vi "Right-Click - Template.vi"() -> ()   [LabVIEW 2011]
doc: "This display template will allow a user to add any numeric or boolean control or indicator to the front panel, and be able to configure it in VeriStand.\n\nSteps:\n1. Add Control / Indicator to the front panel\n2. Right-Click control / indicator and show the Caption (Visible Items >> Caption)\n**Note: No changes on the block diagram are required, however it is advised to put the new controls / indicators in the initialization portion of the code for continuity.\n3. Edit the VI front panel so it only shows the controls and thier captions.\n4. Change the VI window size (File >> VI Properties >> Window Size >> Set to Current)\n5. Save the VI, and Re-build the source distribution\n6. Place new source distribution files here: < Shared Documents >\\ National Instruments\\VeriStand\\Display Templates"
uses:
  <vilib>/NI Veristand/Display Template Support/Display Template Support.llb/cluster_Screen Item Settings.ctl
  <vilib>/NI Veristand/Display Template Support/Display Template Support.llb/cluster_Graph Scale Settings.ctl
  <vilib>/NI Veristand/Display Template Support/Display Template Support.llb/cluster_Graph Plot Settings.ctl
  NationalInstruments.VeriStand.SystemStorage
  <vilib>/NI Veristand/Display Template Support/Display Template Support.llb/enum_Display Template Handler Minimal To Widget Msg.ctl
  <vilib>/NI Veristand/Display Template Support/Display Template Support.llb/enum_Display Template Handler Minimal To Workspace.ctl
  Sub VIs/Custom Data Cluster Control.ctl
  <vilib>/NI Veristand/Display Template Support/Display Template Support.llb/sub_Display Template Handler Custom.vi
  <vilib>/NI Veristand/Execution/Workspace/NI VeriStand - Get Multiple Channel Values.vi
  <vilib>/NI Veristand/Execution/Workspace/NI VeriStand - Set Single Channel Value.vi
  <vilib>/NI Veristand/Execution/Workspace/NI_VS Workspace ExecutionAPI.lvlib
panel:
  in  "NIVS.System Definition Root":refnum<k24>
  in  "NIVS.Gateway IP Address":string
  in  "Ring":u16(ring) items=["Option 1", "Option 2", "Option 3"]
  in  "Boolean":bool
  out "error out":errorcluster
  out "Indicator 2":dbl caption="Numeric"
  out "Indicator 1":dbl caption="Numeric"
  in  "Control 2":dbl caption="Numeric"
  in  "Control 1":dbl caption="Numeric"
  in  "Item.Data":T1
  # "Right-Click a Control or Indicator to configure."
  # "This is needed for the channel selection dialog, do not modify"
  # "This is needed for multi host support, do not modify"
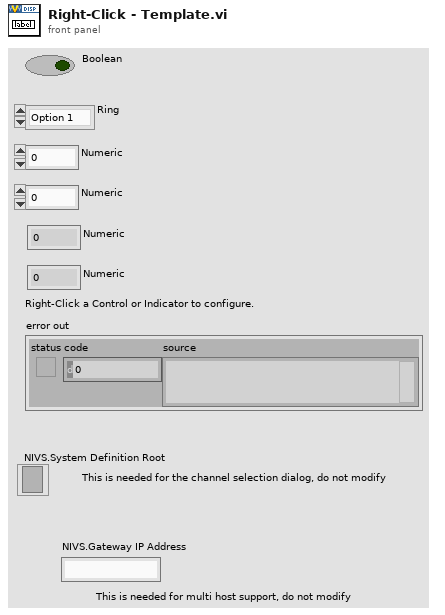
[diagram p1: front panel]
types:
  T1 = typedef "cluster_Screen Item Settings.ctl" = cluster{"Template VI":string, "Position X":i32, "Position Y":i32, "Custom":string, "Show Title Bar":bool, "ID":i32, "Always On Top":bool, "Allow Resize":bool, "Allow Minimize":bool, "Allow Close":bool, "Size to Screen":bool, "Screen.ID":i32, "State":enum16{"Normal", "New"}, "Title":string, "Window Bounds":cluster{"[0]":i16, "[1]":i16, "[2]":i16, "[3]":i16}, "Channel Ref":u64, "Unit":string, "Default Units?":bool, "Flash Limit?":bool, "Color 1":u32, "Color 2":u32, "Color 3":u32, "Color 4":u32, "Bck Color":u32, "Fore Color":u32, "Limit 1":dbl, "Limit 2":dbl, "Limit 3":dbl, "Limit 4":dbl, "Limit Mode 1":i32, "Limit Mode 2":i32, "Limit Mode 3":i32, "Limit Mode 4":i32, "Scale Precision":i32, "Scale Min":dbl, "Scale Max":dbl, "Format":i32, "Precision":i32, "Background Type":i32, "IDs":i32[], "Units":string[], "Labels":string[], "Scale Factor":dbl, "Scale Offset":dbl, "YScale Index":u32[], "XScale":T2, "YScales":T2[], "Plots":T3[], "Update Period":dbl, "History Length":dbl, "My.Ref":refnum<vi>, "Is Control?":bool, "Channel Paths":string[], "Custom Data":variant}
  T2 = typedef "cluster_Graph Scale Settings.ctl" = cluster{"Format":u8, "Precision":u8, "Fit":u8, "Label":string, "Use Default Label":bool, "Label Visible":bool, "Min":dbl, "Max":dbl}
  T3 = typedef "cluster_Graph Plot Settings.ctl" = cluster{"Bar Style":u8, "Fill To":i16, "Fill/PtColor":u32, "Line Style":u8, "Line Width":u8, "Color":u32, "Interp":u8, "Point Style":u8}
  T4 = typedef "enum_Display Template Handler Minimal To Workspace.ctl" = cluster{"Operation":enum16{"SetCustomData", "DeleteItem"}, "Data":variant}
  T5 = typedef "enum_Display Template Handler Minimal To Widget Msg.ctl" = enum16{"Stop", "LaunchConfigDialog"}
  T6 = typedef "Custom Data Cluster Control.ctl" = cluster{"All Refs":refnum<vi>[], "Paths":string[], "Indices":u32[], "NodePathArrays":string[][]}
  T7 = typedef "NI_VS Workspace ExecutionAPI.lvlib/WorkspaceAPI.ctl" = refnum<k24>
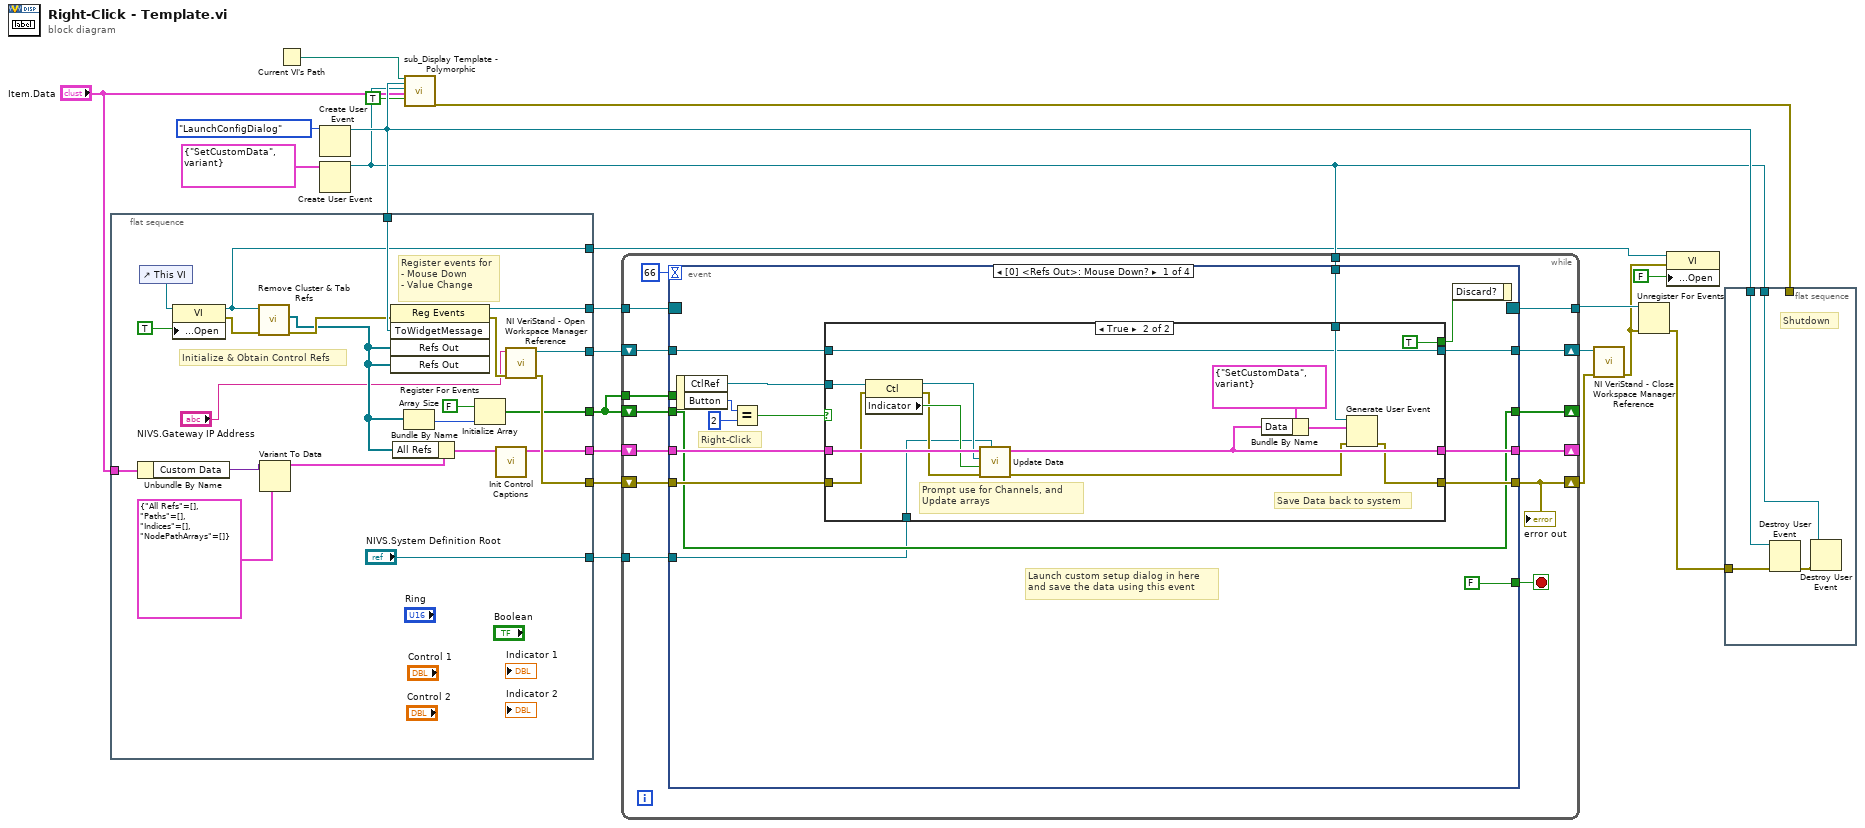
[diagram p0: block diagram]
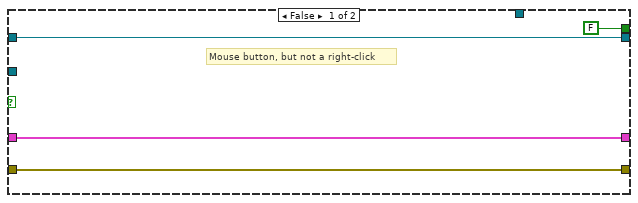
[diagram p2: hidden frame]
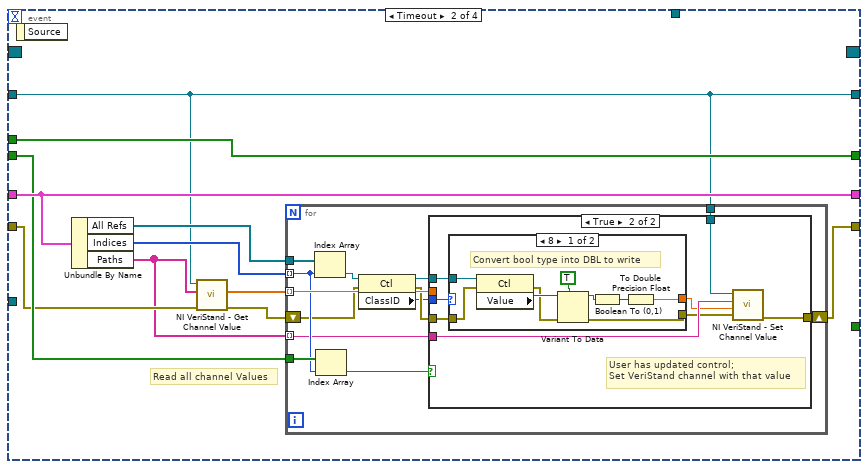
[diagram p3: hidden frame]
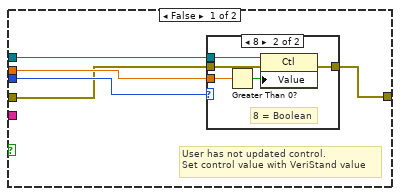
[diagram p4: hidden frame]
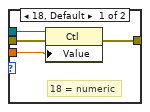
[diagram p5: hidden frame]
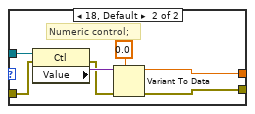
[diagram p6: hidden frame]
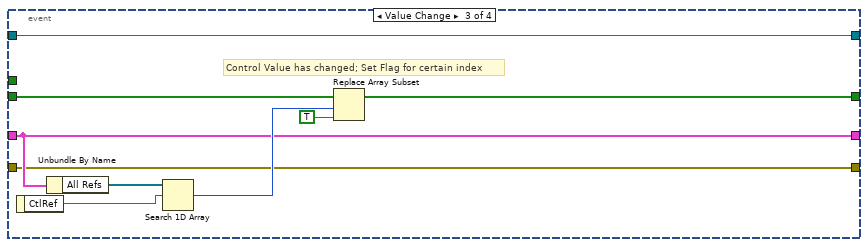
[diagram p7: hidden frame]
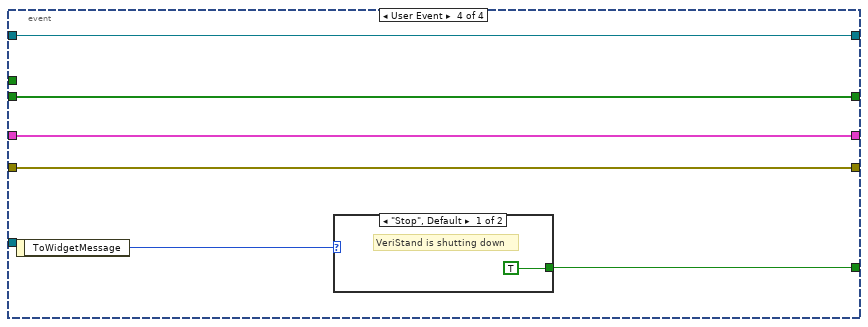
[diagram p8: hidden frame]
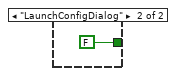
[diagram p9: hidden frame]
diagram:
  n1 = flat-sequence {
    tunnel: w18 -> [w38]
    tunnel: "Item.Data" -> [w43]
    tunnel: [w41] -> w13
    tunnel: [w28] -> w12
    tunnel: [w39] -> w11
    tunnel: [w35] -> w9
    tunnel: [w27] -> w4
    tunnel: [w31] -> w2
    tunnel: ["NIVS.System Definition Root"] -> w1
    frame #0 {
      # "Register events for\n- Mouse Down\n- Value Change"
      # "Initialize & Obtain Control Refs"
      n2 = Unbundle By Name(w43) -> ("Custom Data"=w42:variant)
      n3 = control-ref of="This VI"() -> (w36:refnum<vi>)
      n4 = property class="VI"(reference=w36, "Front Panel.Open"=TRUE ("Front Panel Window:Open")) -> (reference out=w27:refnum<vi>, error out=w26:errorcluster)  [unwired: 1 in]
      n5 = call "Remove Cluster & Tab Refs.vi"("Error In"=w26, "VI Refnum In"=w27) -> ("error out"=w25:errorcluster, "Refs Out"=w24:refnum<vi>[])  [unwired: 7 in, 1 out]
      n6 = Variant To Data(type=T6 {"All Refs"=[], "Paths"=[], "Indices"=[], "NodePathArrays"=[]} ("Custom Data Cluster"), Variant=w42) -> (data=w30:T6)  [unwired: 1 in, 1 out]
      n7 = register-events(error in=w25, w38, w24, w24) -> (reference out=w41:refnum<event-registration>, error out=w40:errorcluster)  [unwired: 1 in]
      n8 = Bundle By Name(cluster=w30, "All Refs"=w24) -> (w29:T6)
      n9 = Array Size(array=w24) -> (size(s)=w32:i32)
      n10 = Initialize Array(FALSE, w32) -> (w31:bool[])
      n11 = call "Init Control Captions.vi"("Custom Data Cluster In"=w29) -> ("Custom Data Cluster Out"=w28:T6)  [unwired: 9 in, 1 out]
      n12 = call <vilib>:"NI VeriStand - Open Workspace Manager Reference.vi"("error in (no error)"=w40, "Gateway IP Address (\"\": localhost)"="NIVS.Gateway IP Address") -> ("error out"=w35:errorcluster, "WorkspaceManager"=w39:T7)  [unwired: 8 in]
    }
  }
  n13 = Current VI's Path() -> (path=w16:path)
  n14 = Create User Event(user event datatype=enum_Display_Template_Handler_Minimal_To_Widget_Msg."LaunchConfigDialog" ("ToWidgetMessage")) -> (user event=w18:refnum<user-event>)  [unwired: 1 in, 1 out]
  n15 = Create User Event(user event datatype=T4 {"Operation"=enum."SetCustomData", "Data"=variant} ("Data")) -> (user event=w10:refnum<user-event>)  [unwired: 1 in, 1 out]
  n16 = call-poly <vilib>:"sub_Display Template - Polymorphic.vi"("Parent.Path"=w16, "ToWidgetEvent"=w18, "ToWorkspace"=w10, "Item.Data"="Item.Data", "Resizable"=TRUE) -> ("error out"=w21:errorcluster)  [unwired: 1 in, 13 out]
  n17 = while {
    tunnel: [w57] -> w19
    tunnel: w13 -> [w56]
    shift-right: [w52] -> _
    shift-left: w12 -> [w55]
    shift-right: [w53] -> w8
    shift-left: w11 -> [w54]
    tunnel: w10 -> [w50]
    shift-right: [w45] -> w7
    shift-left: w9 -> [w49]
    shift-right: [w47] -> _
    shift-left: w2 -> [w48]
    tunnel: w2 -> [w46]
    tunnel: w1 -> [w44]
    stop <- w58 stop-if-true
    n18 = event shown="[0] <Refs Out>: Mouse Down?" {
      selector: w56 -> [_ _ _ _]
      dyn-events: [_ _ _ _] -> w57
      timeout: 66 -> [_ _ _ _]
      tunnel: [FALSE _ _ w168] -> w58
      tunnel: w55 -> [w70 w103 w157 w166]
      tunnel: w54 -> [w69 w93 w155 w165]
      tunnel: [w68 w93 w155 w165] -> w53
      tunnel: [w67 w103 w157 w166] -> w52
      tunnel: w50 -> [w71 _ _ _]
      tunnel: w49 -> [w65 w98 w156 w167]
      tunnel: [w66 w96 w156 w167] -> w45
      tunnel: w48 -> [w60 w99 w161 w164]
      tunnel: [w60 w97 w158 w164] -> w47
      tunnel: w46 -> [_ w97 _ _]
      tunnel: w44 -> [w59 _ _ _]
      event Mouse Down? {
        # "Right-Click"
        # "Launch custom setup dialog in here\nand save the data using this event"
        n19 = event-data() -> ("CtlRef"=w72:refnum<vi>, "Button"=w64:u16)  [unwired: 1 out]
        n20 = Equal?(x=w64, y=u16 2) -> (x = y?=w62:bool)
        n21 = case shown="True" w62 {
          tunnel: w72 -> [_ w92]
          tunnel: w71 -> [_ w91]
          tunnel: w70 -> [w75 w90]
          tunnel: w69 -> [w77 w79]
          tunnel: [w77 w79] -> w68
          tunnel: [w75 w85] -> w67
          tunnel: [w76 w84] -> w66
          tunnel: w65 -> [w76 w83]
          tunnel: [FALSE ("Discard?") TRUE ("Discard?")] -> w61
          tunnel: w59 -> [_ w78]
          frame False {
            # "Mouse button, but not a right-click"
          }
          frame True {
            # "Save Data back to system"
            # "Prompt use for Channels, and \nUpdate arrays"
            n22 = property class="Ctl"(reference=w92, error in=w83) -> (reference out=w89:refnum<vi>, error out=w81:errorcluster, "Indicator"=w88:bool)
            n23 = call "Update Data.vi"("NIVS.System Definition Root"=w78, "Error In"=w81, "Indicator?"=w88, "Control Reference In"=w89, "Custom Data Cluster In"=w90) -> ("error Out"=w80:errorcluster, "Custom Data Cluster Out"=w85:T6)  [unwired: 5 in]
            n24 = Bundle By Name(cluster=T4 {"Operation"=enum."SetCustomData", "Data"=variant} ("event data"), "Data"=w85) -> (w87:T4)
            n25 = Generate User Event(user event=w91, event data cluster=w87, error in=w80) -> (error out=w84:errorcluster)  [unwired: 1 out]
          }
        }
        n26 = event-data("Discard?"=w61) -> ()  [unwired: 1 in, 1 out]
      }
      event Timeout {
        # "Read all channel Values"
        n27 = event-data() -> ()  [unwired: 2 out]
        n28 = Unbundle By Name(w103) -> ("All Refs"=w102:refnum<vi>[], "Indices"=w95:u32[], "Paths"=w94:string[])
        n29 = call-poly <vilib>:"NI VeriStand - Get Channel Value.vi"("error in (no error)"=w98, "Channels"=w94, "WorkspaceManager in"=w93) -> ("error out"=w100:errorcluster, "Values"=w101:dbl[])  [unwired: 6 in, 1 out]
        n30 = for {
          tunnel: w95 -> [w111] mode=indexing
          tunnel: w101 -> [w116] mode=indexing
          shift-right: [w115] -> w96
          shift-left: w100 -> [w106]
          tunnel: w102 -> [w114]
          tunnel: w99 -> [w112]
          tunnel: w94 -> [w110] mode=indexing
          tunnel: w93 -> [w109]
          n31 = Index Array(array=w114, index=w111) -> (element=w108:refnum<vi>)
          n32 = Index Array(array=w112, index=w111) -> (element=w113:bool)
          n33 = property class="Ctl"(reference=w108, error in=w106) -> (reference out=w107:refnum<vi>, error out=w105:errorcluster, "ClassID"=w104:u32)
          n34 = case shown="True" w113 {
            tunnel: w116 -> [w120 _]
            tunnel: w105 -> [w117 w133]
            tunnel: [w121 w137] -> w115
            tunnel: w107 -> [w118 w134]
            tunnel: w109 -> [_ w138]
            tunnel: w110 -> [_ w136]
            tunnel: w104 -> [w119 w135]
            frame False {
              # "User has not updated control. \nSet control value with VeriStand value"
              n35 = case shown="8" w119 {
                tunnel: [w123 w130] -> w121
                tunnel: w117 -> [w124 w129]
                tunnel: w118 -> [w125 w128]
                tunnel: w120 -> [w122 w127]
                frame 18, Default {
                  # "18 = numeric"
                  n36 = property class="Ctl"(reference=w125, error in=w124, "Value"=w122) -> (error out=w123:errorcluster)  [unwired: 1 out]
                }
                frame 8 {
                  # "8 = Boolean"
                  n37 = Greater Than 0?(x=w127) -> (x > 0?=w126:bool)
                  n38 = property class="Ctl"(reference=w128, error in=w129, "Value"=w126) -> (error out=w130:errorcluster)  [unwired: 1 out]
                }
              }
            }
            frame True {
              # "User has updated control; \nSet VeriStand channel with that value"
              n39 = case shown="8" w135 {
                tunnel: w134 -> [w142 w153]
                tunnel: w133 -> [w141 w152]
                tunnel: [w139 w149] -> w132
                tunnel: [w143 w148] -> w131
                frame 8 {
                  # "Convert bool type into DBL to write"
                  n40 = property class="Ctl"(reference=w142, error in=w141) -> (error out=w140:errorcluster, "Value"=w144:variant)  [unwired: 1 out]
                  n41 = Variant To Data(error in=w140, type=TRUE, Variant=w144) -> (data=w146:bool, error out=w139:errorcluster)
                  n42 = Boolean To (0,1)(Boolean=w146) -> (0, 1=w147:i16)
                  n43 = To Double Precision Float(number=w147) -> (double precision float=w143:dbl)
                }
                frame 18, Default {
                  # "Numeric control;"
                  n44 = property class="Ctl"(reference=w153, error in=w152) -> (error out=w150:errorcluster, "Value"=w154:variant)  [unwired: 1 out]
                  n45 = Variant To Data(error in=w150, type=0.0, Variant=w154) -> (data=w148:dbl, error out=w149:errorcluster)
                }
              }
              n46 = call-poly <vilib>:"NI VeriStand - Set Channel Value.vi"("error in (no error)"=w132, "Value"=w131, "Channel"=w136, "WorkspaceManager in"=w138) -> ("error out"=w137:errorcluster)  [unwired: 6 in, 1 out]
            }
          }
        }
      }
      event Value Change {
        # "Control Value has changed; Set Flag for certain index"
        n47 = event-data() -> ("CtlRef"=w162:refnum<vi>)  [unwired: 1 out]
        n48 = Unbundle By Name(w157) -> ("All Refs"=w163:refnum<vi>[])
        n49 = Search 1D Array(1D array=w163, element=w162) -> (index of element=w160:i32)  [unwired: 1 in]
        n50 = Replace Array Subset(array=w161, new element=TRUE ("new element/subarray"), index=w160) -> (w158:bool[])
      }
      event User Event {
        n51 = event-data() -> ("ToWidgetMessage"=w169:T5)  [unwired: 1 out]
        n52 = case shown="\"Stop\", Default" w169 {
          tunnel: [TRUE FALSE] -> w168
          frame "Stop", Default {
            # "VeriStand is shutting down"
          }
          frame "LaunchConfigDialog" {
          }
        }
      }
    }
    "error out" <- w45
  }
  n53 = call <vilib>:"NI VeriStand - Close Workspace Manager Reference.vi"("error in (no error)"=w7, "WorkspaceManager"=w8) -> ("error out"=w5:errorcluster)  [unwired: 9 in]
  n54 = Unregister For Events(event registration refnum=w19, error in=w5) -> (error out=w6:errorcluster)
  n55 = property class="VI"(reference=w4, error in=w5, "Front Panel.Open"=FALSE ("Front Panel Window:Open")) -> ()  [unwired: 2 out]
  n56 = flat-sequence {
    tunnel: w21 -> [_]
    tunnel: w6 -> [w174]
    tunnel: w18 -> [w175]
    tunnel: w10 -> [w172]
    frame #0 {
      # "Shutdown"
      n57 = Destroy User Event(user event=w175, error in=w174) -> (error out=w173:errorcluster)
      n58 = Destroy User Event(user event=w172, error in=w173) -> ()  [unwired: 1 out]
    }
  }
